vi "PH_ImageOperator.GaussFit.vi"(0 "Index":dbl[](array[numeric]) format="%0.2f", 1 "Standard Deviation":dbl[](array[numeric]) format="%0.2f", 5 "Trace":dbl[](array[numeric]) format="%0.2f", 7 "No Offset?":bool, 9 "Initial Guess Coefficients":dbl[](array[numeric]) format="%0.2f", 11 "max iteration":i32=200, 12 "Order of GAUSSian function":i32) -> (4 "Best Fit Coefficients":dbl[](array[numeric]) format="%0.2f", 6 "Best Fit":dbl[](array[numeric]) format="%0.2f", 8 "Covariance":dbl[][](array[numeric]) format="%0.2f", 10 "mse":dbl format="%0.4e", 15 "error":i32)   [LabVIEW 2014, in "PH_ImageOperator.lvlib"]
doc: "Uses the Levenberg-Marquardt algorithm to determine the different GAUSS function fits to the traces."
uses:
  PH_ImageOperator.lvlib
  <vilib>/Analysis/baseanly.llb/Real Inverse Matrix.vi
  <vilib>/Analysis/NI_AALPro.lvlib
  <vilib>/Analysis/NI_AALBase.lvlib
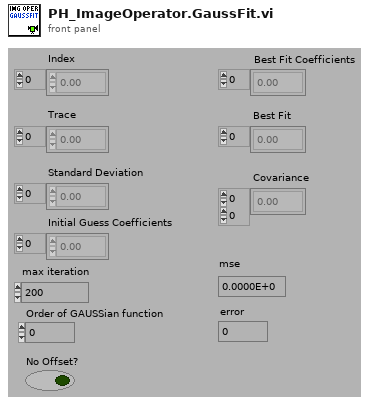
[diagram p1: front panel]
types:
  T1 = typedef "NI_Matrix.lvlib/RealMatrix.ctl" = dbl[][]
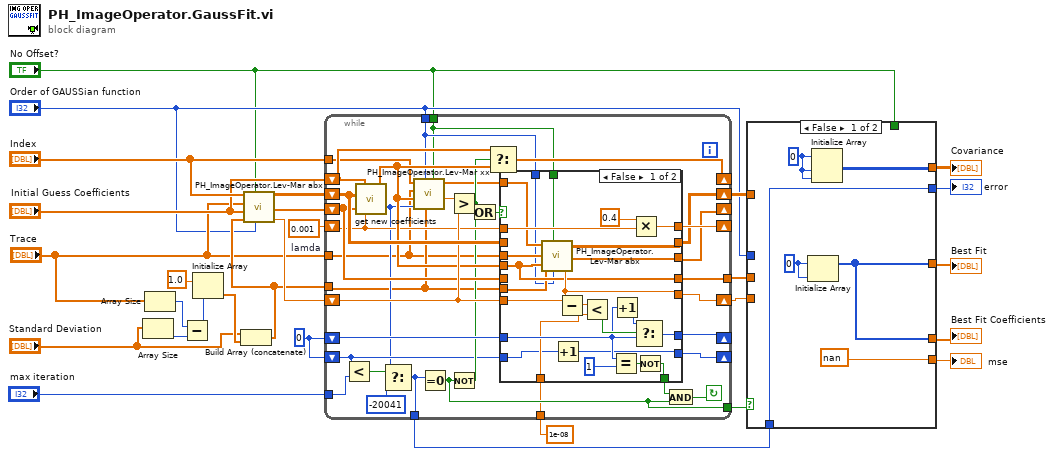
[diagram p0: block diagram]
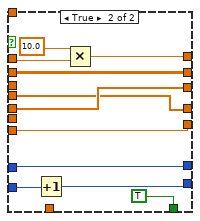
[diagram p2: hidden frame]
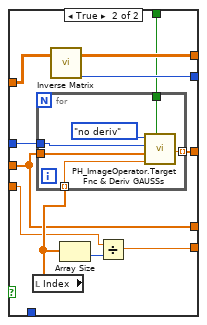
[diagram p3: hidden frame]
diagram:
  w18 = 0
  w27 = 0.001  # lamda
  n1 = Array Size(array="Standard Deviation") -> (size(s)=w8:i32)
  n2 = Array Size(array="Trace") -> (size(s)=w9:i32)
  n3 = Subtract(x=w9, y=w8) -> (x-y=w7:i32)
  n4 = Initialize Array(1.0, w7) -> (w6:dbl[])
  n5 = Build Array (concatenate)("Standard Deviation", w6) -> (w4:dbl[])
  n6 = call "PH_ImageOperator.Lev-Mar abx.vi"("Order of GAUSSian function"="Order of GAUSSian function", "No Offset?"="No Offset?", "Standard Deviation"=w4, "Coefficients"="Initial Guess Coefficients", "Y"="Trace", "X"="Index") -> ("chiSqr"=w25:dbl, "Beta"=w26:dbl[], "Alpha"=w28:dbl[][])  [unwired: 1 in]
  n7 = while {
    tunnel: "Index" -> [w32]
    tunnel: "Trace" -> [w34]
    tunnel: [w35] -> w11
    tunnel: "max iteration" -> [w37]
    tunnel: w4 -> [w36]
    shift-left: w18 -> [w41]
    shift-right: [w42] -> _
    tunnel: 1e-08 -> [w46]
    tunnel: [w47] -> w20
    tunnel: [w50] -> w23
    shift-left: w18 -> [w55]
    shift-right: [w54] -> _
    shift-left: w25 -> [w56]
    shift-right: [w57] -> w24
    shift-left: w26 -> [w53]
    shift-right: [w58] -> _
    shift-left: w28 -> [w59]
    shift-right: [w60] -> w10
    shift-left: "Initial Guess Coefficients" -> [w33]
    shift-right: [w61] -> _
    shift-left: w27 -> [w51]
    shift-right: [w62] -> _
    tunnel: "Order of GAUSSian function" -> [w31]
    tunnel: "No Offset?" -> [w30]
    stop <- w49 continue-if-true
    n8 = Less?(x=w41, y=w37) -> (x < y?=w40:bool)
    n9 = call <vilib>:"get new coefficients.vi"("lamda"=w51, "Beta"=w53, "Alpha"=w59, "Coefficients"=w33) -> ("error"=w38:i32, "New Coefficients"=w52:dbl[])
    n10 = Select(t=w38, s=w40, f=-20041) -> (s? t:f=w35:i32)
    n11 = call "PH_ImageOperator.Lev-Mar xx.vi"("No Offset?"=w30, "Standard Deviation"=w36, "Order of GAUSSian function"=w31, "error"=w38, "Coefficients"=w52, "Y"=w34, "X"=w32) -> ("chiSqr"=w63:dbl)  [unwired: 3 in]
    n12 = Equal To 0?(x=w35) -> (x = 0?=w47:bool)
    n13 = Greater?(x=w63, y=w56) -> (0:w44:bool)
    n14 = Not(x=w47) -> (.not. x?=w43:bool)
    n15 = Or(x=w44, y=w43) -> (x .or. y?=w45:bool)
    n16 = Select(t=w33, s=w44, f=w52) -> (s? t:f=w61:dbl[])
    n17 = case shown="False" w45 {
      tunnel: w51 -> [w86 w97]
      tunnel: [w85 w96] -> w62
      tunnel: [w84 w95] -> w60
      tunnel: w59 -> [_ w95]
      tunnel: [w83 w91] -> w58
      tunnel: [w82 w94] -> w57
      tunnel: w56 -> [w81 w94]
      tunnel: w55 -> [w76 w93]
      tunnel: [w77 w93] -> w54
      tunnel: [w73 TRUE] -> w48
      tunnel: w52 -> [w70 w90]
      tunnel: w53 -> [_ w91]
      tunnel: [w70 w90] -> w50
      tunnel: w46 -> [w72 _]
      tunnel: [w68 w89] -> w42
      tunnel: w41 -> [w71 w88]
      tunnel: w36 -> [w69 _]
      tunnel: w32 -> [w67 _]
      tunnel: w34 -> [w66 _]
      tunnel: w31 -> [w65 _]
      tunnel: w30 -> [w64 _]
      frame False {
        n18 = call "PH_ImageOperator.Lev-Mar abx.vi"("Order of GAUSSian function"=w65, "No Offset?"=w64, "Standard Deviation"=w69, "Coefficients"=w70, "Y"=w66, "X"=w67) -> ("chiSqr"=w82:dbl, "Beta"=w83:dbl[], "Alpha"=w84:dbl[][])  [unwired: 1 in]
        n19 = Increment(x=w71) -> (x+1=w68:i32)
        n20 = Subtract(x=w81, y=w82) -> (x-y=w80:dbl)
        n21 = Less?(x=w80, y=w72) -> (x < y?=w79:bool)
        n22 = Equal?(x=w76, y=1) -> (x = y?=w74:bool)
        n23 = Increment(x=w76) -> (x+1=w78:i32)
        n24 = Multiply(x=0.4, y=w86) -> (x*y=w85:dbl)
        n25 = Select(t=w78, s=w79, f=w76) -> (s? t:f=w77:i32)
        n26 = Not(x=w74) -> (.not. x?=w73:bool)
      }
      frame True {
        n27 = Increment(x=w88) -> (x+1=w89:i32)
        n28 = Multiply(x=10.0, y=w97) -> (x*y=w96:dbl)
      }
    }
    n29 = And(x=w48, y=w47) -> (x .and. y?=w49:bool)
  }
  n30 = case shown="False" w20 {
    tunnel: w23 -> [_ w111]
    tunnel: [w102 w111] -> w22
    tunnel: [nan w115] -> w21
    tunnel: [w102 w112] -> w14
    tunnel: w24 -> [_ w110]
    tunnel: [w100 w109] -> w13
    tunnel: [w99 w108] -> w12
    tunnel: w11 -> [w99 _]
    tunnel: w10 -> [_ w107]
    tunnel: "Order of GAUSSian function" -> [_ w106]
    tunnel: "No Offset?" -> [_ w105]
    frame False {
      w101 = 0
      w104 = 0
      n31 = Initialize Array(w104, w104) -> (w102:i32[])
      n32 = Initialize Array(w101, w101, w101) -> (w100:i32[][])
    }
    frame True {
      n33 = local read "Index"() -> (w114:dbl[])
      n34 = for {
        tunnel: w111 -> [w120]
        tunnel: [w119] -> w112 mode=indexing
        tunnel: w114 -> [w121] mode=indexing
        tunnel: w106 -> [w117]
        tunnel: w105 -> [w116]
        n35 = call "PH_ImageOperator.Target Fnc & Deriv GAUSSs.vi"("Flag"=enum16{"no deriv", "deriv"}."no deriv", "Order of GAUSSian function"=w117, "Coefficients"=w120, "X"=w121, "No Offset?"=w116) -> ("Y"=w119:dbl)  [unwired: 1 out]
      }
      n36 = call-poly <vilib>:"Inverse Matrix.vi"("Input Matrix"=w107) -> ("error"=w108:i32, "Inverse Matrix"=w109:T1)  [unwired: 1 in]
      n37 = Array Size(array=w114) -> (size(s)=w113:i32)
      n38 = Divide(x=w110, y=w113) -> (x/y=w115:dbl)
    }
  }
  "mse" <- w21
  "Best Fit Coefficients" <- w22
  "Best Fit" <- w14
  "error" <- w12
  "Covariance" <- w13
